vi "Channel A and or B (Demo).vi"(0 "Level":dbl format="%.2f", 1 "Frequency":dbl format="%.2f", 2 "Slope":bool, 3 "Source":bool, 4 "Select Channel":u32 max=2 step=1, 5 "No. Points":i32) -> (6 "Waveform 1 Out":dbl[](array[numeric]) format="%.2f", 7 "Noise":dbl[](array[numeric]) format="%.2f", 8 "Waveform 2 Out":dbl[](array[numeric]) format="%.2f")   [LabVIEW 2009]
doc: "This VI is used to simulate signals from an oscilloscope on channels A, B, or both A&B. This VI simulates a GPIB instrument driver."
uses:
  <vilib>/Analysis/NI_AALBase.lvlib
panel:
  # "POS\nNEG"
  # "CH B\nEXT"
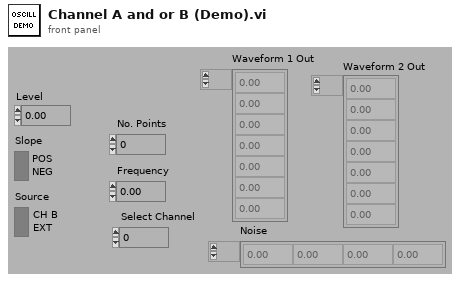
[diagram p1: front panel]
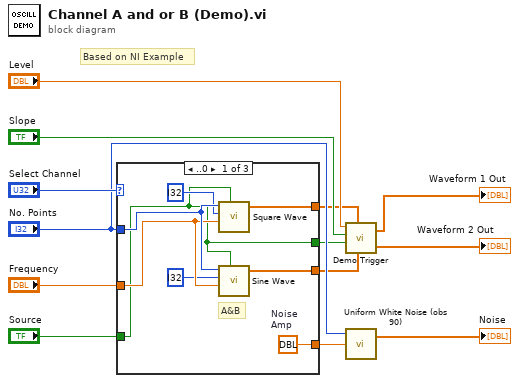
[diagram p0: block diagram]
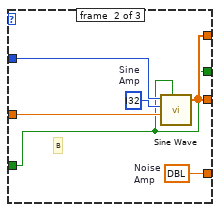
[diagram p2: hidden frame]
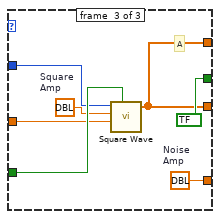
[diagram p3: hidden frame]
diagram:
  # "Based on NI Example"
  n1 = case shown="..0" "Select Channel" {
    tunnel: "Source" -> [w14 w22 w34]
    tunnel: "No. Points" -> [w20 w27 w33]
    tunnel: [w21 w25 w31] -> w8
    tunnel: "Frequency" -> [w19 w24 w30]
    tunnel: [w14 w22 bool ?] -> w5
    tunnel: [w15 w23 w28] -> w4
    tunnel: [w16 w23 w28] -> w3
    frame #0 {
      w21 = dbl ?  # Noise Amp
      # "A&B"
      n2 = call <vilib>:"Square Wave.vi"("samples"=w20, "reset phase"=w14, "amplitude"=i32 ?, "frequency"=w19) -> ("square wave"=w15:dbl[])  [unwired: 2 in, 2 out]
      n3 = call <vilib>:"Sine Wave.vi"("samples"=w20, "amplitude"=i32 ?, "frequency"=w19, "reset phase"=w14) -> ("sine wave"=w16:dbl[])  [unwired: 1 in, 2 out]
    }
    frame #1 {
      w26 = i32 ?  # Sine Amp
      w25 = dbl ?  # Noise Amp
      # "B"
      n4 = call <vilib>:"Sine Wave.vi"("samples"=w27, "amplitude"=w26, "frequency"=w24, "reset phase"=w22) -> ("sine wave"=w23:dbl[])  [unwired: 1 in, 2 out]
    }
    frame #2 {
      w32 = dbl ?  # Square Amp
      w31 = dbl ?  # Noise Amp
      # "A"
      n5 = call <vilib>:"Square Wave.vi"("samples"=w33, "reset phase"=w34, "amplitude"=w32, "frequency"=w30) -> ("square wave"=w28:dbl[])  [unwired: 2 in, 2 out]
    }
  }
  n6 = call "Demo Trigger.vi"("Waveform 2 In"=w3, "Waveform 1 In"=w4, "Source"=w5, "Slope"="Slope", "Level"="Level") -> ("Waveform 2 Out"=→"Waveform 2 Out":dbl[], "Waveform 1 Out"=→"Waveform 1 Out":dbl[])  [unwired: 1 in]
  n7 = call <vilib>:"Uniform White Noise (obs 90).vi"("amplitude"=w8, "samples"="No. Points") -> ("uniform white noise"=→"Noise":dbl[])  [unwired: 1 in, 1 out]
